vi "SIUnitConverter.vi"(11 "Number":dbl) -> (2 "SI prefix":string, 3 "SI power":dbl)   [LabVIEW 2024]
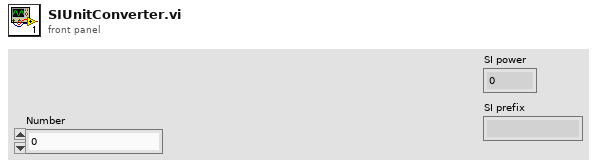
[diagram p1: front panel]
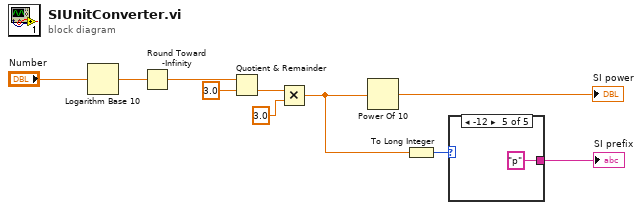
[diagram p0: block diagram]
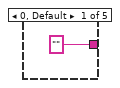
[diagram p2: hidden frame]
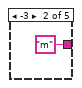
[diagram p3: hidden frame]
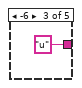
[diagram p4: hidden frame]
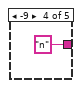
[diagram p5: hidden frame]
diagram:
  n1 = Logarithm Base 10(1:"Number") -> (0:w9:dbl)
  n2 = Round Toward -Infinity(1:w9) -> (0:w8:dbl)
  n3 = Quotient & Remainder(x=w8, y=3.0) -> (floor(x/y)=w6:dbl)  [unwired: 1 out]
  n4 = Multiply(x=w6, y=3.0) -> (x*y=w2:dbl)
  n5 = Power Of 10(x=w2) -> (10^x=→"SI power":dbl)
  n6 = To Long Integer(number=w2) -> (32bit integer=w3:i32)
  n7 = case shown="-12" w3 {
    tunnel: ["" "m" "u" "n" "p"] -> w1
    frame 0, Default {
    }
    frame -3 {
    }
    frame -6 {
    }
    frame -9 {
    }
    frame -12 {
    }
  }
  "SI prefix" <- w1
